vi "CalcMagnitude.vi"(8 "input valid":bool=TRUE, 11 "Data in":fxp<+/-,16,14>[](array[numeric])=[0.0, 0.0, 0.0, 0.0]) -> (0 "output valid":bool, 2 "Amp1":fxp<+,16,14>, 3 "Amp0":fxp<+,16,14>, 5 "Q0 in":fxp<+/-,16,14>, 7 "I0 in":fxp<+/-,16,14>)   [LabVIEW 2013]
uses:
  <vilib>/rvi/FXPMathLib/FxpSqrt/subVIs/nifxpmath_Sqrt_SimConfig.ctl
  <vilib>/fxp/LVFixedPointOverflowPolicyTypeDef.ctl
  <vilib>/rvi/FXPMathLib/FxpSqrt/simVIs/DllSqrtTemp_sub.vi
  <vilib>/rvi/FXPMathLib/FxpSqrt/XNode/nifxpmath_Sqrt.xnode
  <vilib>/rvi/FXPMathLib/FxpAdd/XNode/nifxpmath_Add.xnode
  <vilib>/rvi/FXPMathLib/FxpMul/XNode/nifxpmath_Multiplier.xnode
  <vilib>/rvi/FXPMathLib/sim/FxpSim.dll
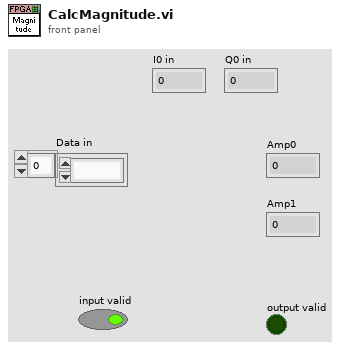
[diagram p1: front panel]
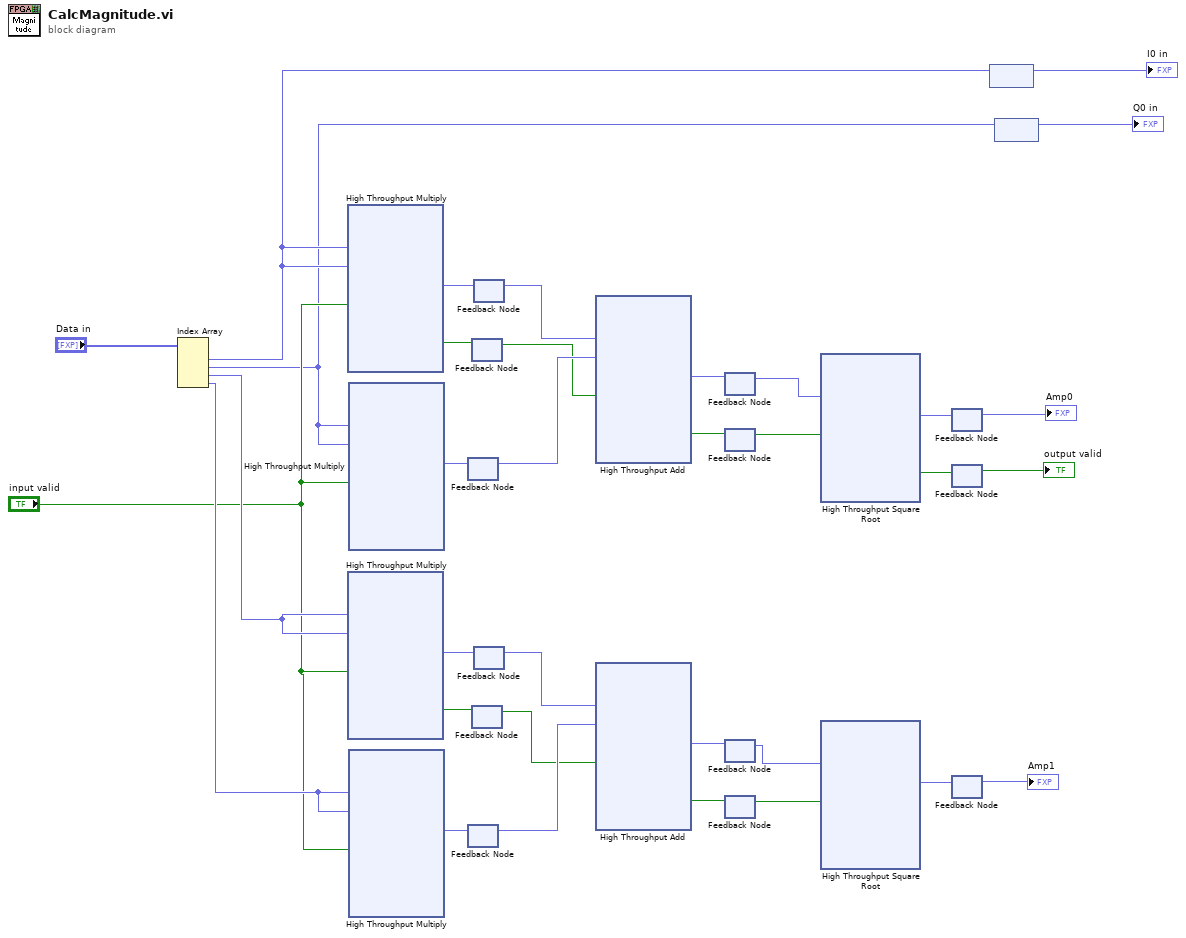
[diagram p0: block diagram]
diagram:
  n1 = Index Array(array="Data in") -> (element #1=w6:fxp<+/-,16,14>, element #2=w2:fxp<+/-,16,14>, element #3=w16:fxp<+/-,16,14>, element #4=w15:fxp<+/-,16,14>)  [unwired: 4 in]
  n2 = xnode "High Throughput Multiply"("x"=w6, "y"=w6, "input valid"="input valid") -> ("x*y"=w9:fxp<+,32,28>, "output valid"=w7:bool)  [unwired: 1 in, 1 out]
  n3 = xnode "High Throughput Multiply"("x"=w16, "y"=w16, "input valid"="input valid") -> ("x*y"=w19:fxp<+,32,28>, "output valid"=w17:bool)  [unwired: 1 in, 1 out]
  n4 = xnode "High Throughput Multiply"("x"=w2, "y"=w2, "input valid"="input valid") -> ("x*y"=w33:fxp<+,32,28>)  [unwired: 1 in, 2 out]
  n5 = xnode "High Throughput Multiply"("x"=w15, "y"=w15, "input valid"="input valid") -> ("x*y"=w21:fxp<+,32,28>)  [unwired: 1 in, 2 out]
  n6 = feedback #1() -> (w32:fxp<+,32,28>)  [unwired: 1 in]
  n7 = feedback-in #1(w33) -> ()
  n8 = feedback #2() -> (w22:fxp<+,32,28>)  [unwired: 1 in]
  n9 = feedback-in #2(w21) -> ()
  n10 = feedback-in #3(w7) -> ()
  n11 = feedback #3() -> (w8:bool)  [unwired: 1 in]
  n12 = feedback #4() -> (w18:bool)  [unwired: 1 in]
  n13 = feedback-in #4(w17) -> ()
  n14 = feedback #5() -> (w10:fxp<+,32,28>)  [unwired: 1 in]
  n15 = feedback-in #5(w9) -> ()
  n16 = feedback #6() -> (w20:fxp<+,32,28>)  [unwired: 1 in]
  n17 = feedback-in #6(w19) -> ()
  n18 = xnode "High Throughput Add"("x"=w10, "y"=w32, "input valid"=w8) -> ("x+y"=w30:fxp<+,32,28>, "output valid"=w31:bool)  [unwired: 1 in, 1 out]
  n19 = xnode "High Throughput Add"("x"=w20, "y"=w22, "input valid"=w18) -> ("x+y"=w25:fxp<+,32,28>, "output valid"=w23:bool)  [unwired: 1 in, 1 out]
  n20 = feedback #7() -> (w29:fxp<+,32,28>)  [unwired: 1 in]
  n21 = feedback-in #7(w30) -> ()
  n22 = feedback #8() -> (w13:bool)  [unwired: 1 in]
  n23 = feedback-in #8(w31) -> ()
  n24 = feedback #9() -> (w26:fxp<+,32,28>)  [unwired: 1 in]
  n25 = feedback-in #9(w25) -> ()
  n26 = feedback #10() -> (w24:bool)  [unwired: 1 in]
  n27 = feedback-in #10(w23) -> ()
  n28 = xnode "High Throughput Square Root"("x"=w29, "input valid"=w13) -> ("sqrt(x)"=w28:fxp<+,16,14>, "output valid"=w11:bool)  [unwired: 1 in, 1 out]
  n29 = xnode "High Throughput Square Root"("x"=w26, "input valid"=w24) -> ("sqrt(x)"=w27:fxp<+,16,14>)  [unwired: 1 in, 2 out]
  n30 = feedback #11() -> (→"Amp0":fxp<+,16,14>)  [unwired: 1 in]
  n31 = feedback-in #11(w28) -> ()
  n32 = feedback #12() -> (→"output valid":bool)  [unwired: 1 in]
  n33 = feedback-in #12(w11) -> ()
  n34 = feedback #13() -> (→"Amp1":fxp<+,16,14>)  [unwired: 1 in]
  n35 = feedback-in #13(w27) -> ()
  n36 = feedback #14() -> (→"I0 in":fxp<+/-,16,14>)  [unwired: 1 in]
  n37 = feedback-in #14(w6) -> ()
  n38 = feedback #15() -> (→"Q0 in":fxp<+/-,16,14>)  [unwired: 1 in]
  n39 = feedback-in #15(w2) -> ()
